vi "RIOPXIStar.vi"(11 "FPGA Name":string) -> (3 "PXI_Star":string)   [LabVIEW 2015]
doc: "Takes a MAX device Name and dentifies the Slot of the device and outputs the PXI_Star line the device is connected to in the chasis.\nThis VI is for PXIe chassis not PXI chassis.\n\nThe numbering is as follows:\nSlot 2 PXI_Star0\nSlot 3 PXI_Star1\nSlot 4 (Sync Card)\nSlot 5 PXI_star_3\nSlot 6 PXI_Star_4\nSlot 7 PXI_Star_5\nSlot8 PXI_Star_6"
panel:
  out "decimal integer string":string
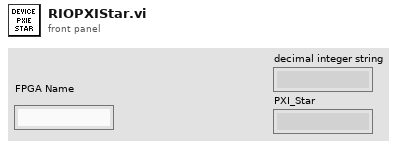
[diagram p1: front panel]
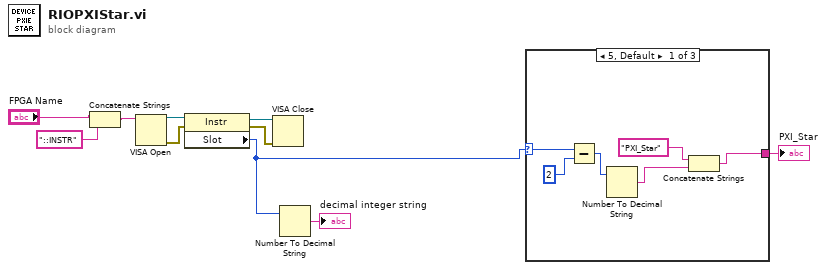
[diagram p0: block diagram]
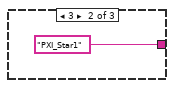
[diagram p2: hidden frame]
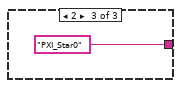
[diagram p3: hidden frame]
diagram:
  n1 = Concatenate Strings("FPGA Name", "::INSTR" ("string")) -> (w8:string)
  n2 = VISA Open(VISA resource name=w8) -> (VISA resource name=w7:refnum<visa-resource-name>, error out=w4:errorcluster)  [unwired: 4 in]
  n3 = property class="Instr"(reference=w7, error in=w4) -> (reference out=w6:refnum<visa-resource-name>, error out=w5:errorcluster, "Slot"=w2:i16)
  n4 = VISA Close(VISA resource name=w6, error in (no error)=w5) -> ()  [unwired: 1 out]
  n5 = Number To Decimal String(number=w2) -> (decimal integer string=→"decimal integer string":string)  [unwired: 1 in]
  n6 = case shown="5, Default" w2 {
    selector: w2 -> [w15 _ _]
    tunnel: [w11 "PXI_Star1" "PXI_Star0"] -> w1
    frame 5, Default {
      n7 = Subtract(x=w15, y=i16 2) -> (x-y=w13:i16)
      n8 = Number To Decimal String(number=w13) -> (decimal integer string=w12:string)  [unwired: 1 in]
      n9 = Concatenate Strings("PXI_Star", w12) -> (w11:string)
    }
    frame 3 {
    }
    frame 2 {
    }
  }
  "PXI_Star" <- w1
